vi "ToPython.vi"() -> ()   [LabVIEW 2019]
panel:
  out "error out":errorcluster
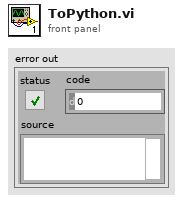
[diagram p1: front panel]
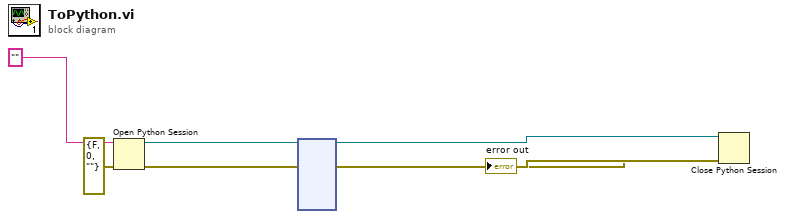
[diagram p0: block diagram]
diagram:
  n1 = Open Python Session(python version="" ("Python version"), 3:errorcluster {"status"=FALSE, "code"=0, "source"=""} ("error in (no error)")) -> (session out=w4:refnum<k35>, error out=w5:errorcluster)  [unwired: 1 in]
  n2 = node(w4, w5) -> (w3:refnum<k35>, w2:errorcluster)  [unwired: 12 in, 2 out]
  n3 = Close Python Session(session in=w3, error in=w2) -> (11:→"error out":errorcluster)
